vi "Rising Edge 2.vi"(1 "Button Pressed?":bool) -> (0 "Bool Output":bool)   [LabVIEW 2015]
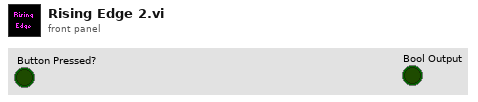
[diagram p1: front panel]
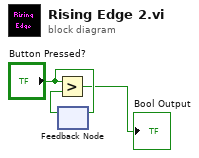
[diagram p0: block diagram]
diagram:
  n1 = feedback-in #1("Button Pressed?") -> ()
  n2 = feedback #1() -> (w3:bool)  [unwired: 1 in]
  n3 = Greater?(x="Button Pressed?", y=w3) -> (0:→"Bool Output":bool)
